vi "1. HelloWorld.vi"() -> ()   [LabVIEW 2011]
panel:
  in  "Disarm":bool
  in  "Arm":bool
  out "OpenSF Error":errorcluster
  out "WriteSF Error":errorcluster
  in  "emergency break":bool
  in  "Destination Id":u16=1
  in  "ServoPositions":T1={"Throttle"=0, "Pitch"=64, "Roll"=64, "Yaw"=64, "Mode"=0, "Data5"=100, "Data6"=100, "Data7"=100}
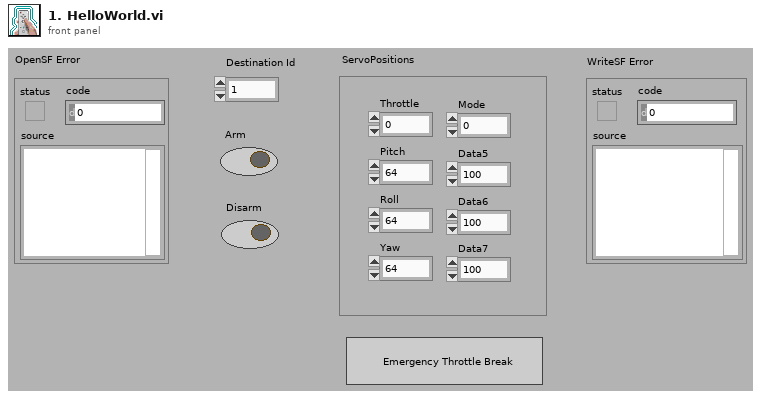
[diagram p1: front panel]
types:
  T1 = cluster{"Throttle":u8, "Pitch":u8, "Roll":u8, "Yaw":u8, "Mode":u8, "Data5":u8, "Data6":u8, "Data7":u8}
  T2 = cluster{"Data0":u8, "Data1":u8, "Data2":u8, "Data3":u8, "Data4":u8, "Data5":u8, "Data6":u8, "Data7":u8}
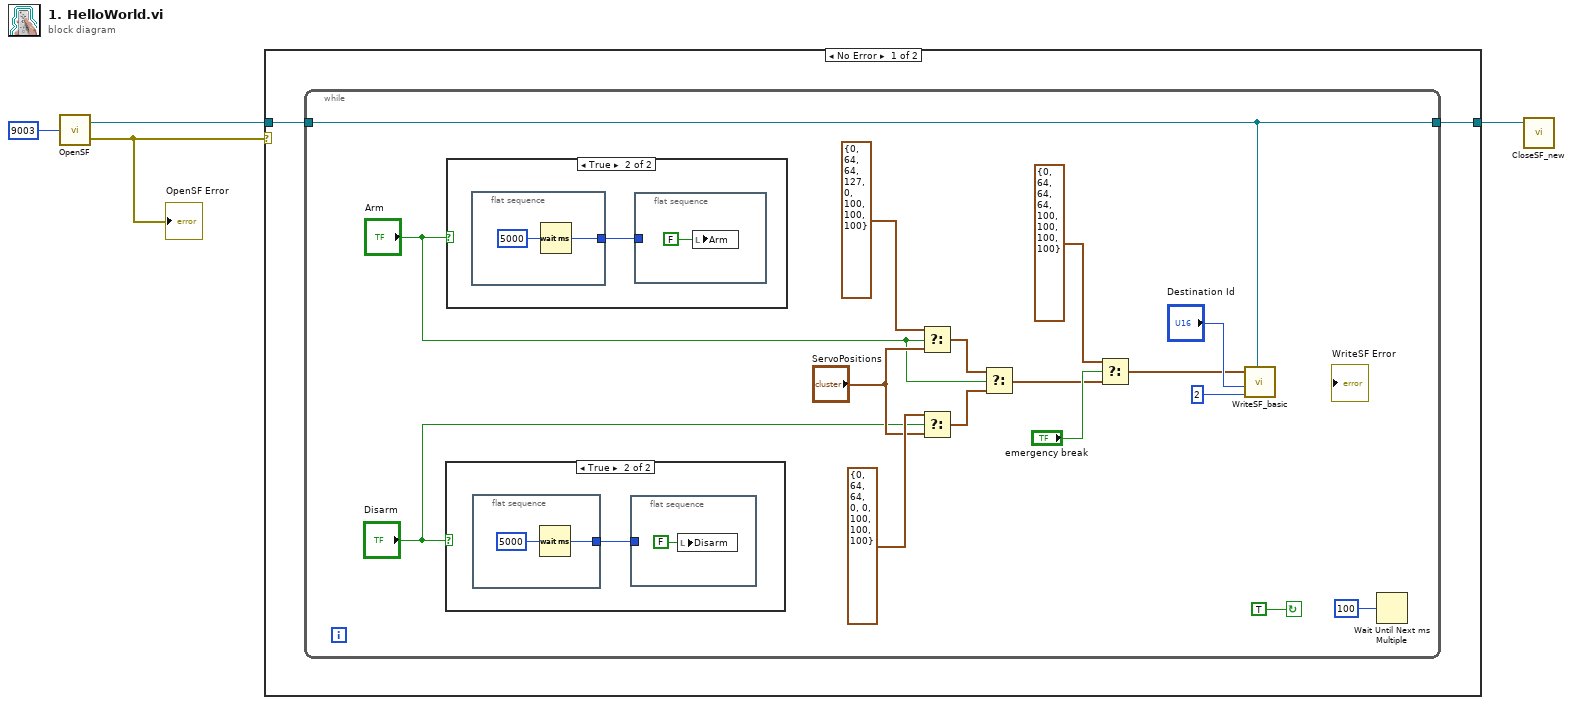
[diagram p0: block diagram]
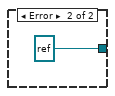
[diagram p4: hidden frame]
diagram:
  n1 = call "OpenSF.vi"("Port number"=u16 9003 ("Port Number")) -> ("connection ID"=w2:refnum<k5>, "Error out"=w3:errorcluster)
  "OpenSF Error" <- w3
  n2 = case shown="No Error" w3 {
    tunnel: w2 -> [w6 _]
    tunnel: [w5 refnum<k5> refnum ("connection ID")] -> w1
    frame No Error {
      n3 = while {
        tunnel: w6 -> [w9]
        tunnel: [w9] -> w5
        stop <- TRUE continue-if-true
        n4 = case shown="True" "Disarm" {
          frame False {
          }
          frame True {
            n5 = flat-sequence {
              tunnel: [w25] -> w23
              frame #0 {
                n6 = Wait (ms)(milliseconds to wait=u32 5000) -> (millisecond timer value=w25:u32)
              }
            }
            n7 = flat-sequence {
              tunnel: w23 -> [_]
              frame #0 {
                n8 = local write "Disarm"(FALSE ("Arm")) -> ()
              }
            }
          }
        }
        n9 = case shown="True" "Arm" {
          frame False {
          }
          frame True {
            n10 = flat-sequence {
              tunnel: [w29] -> w27
              frame #0 {
                n11 = Wait (ms)(milliseconds to wait=u32 5000) -> (millisecond timer value=w29:u32)
              }
            }
            n12 = flat-sequence {
              tunnel: w27 -> [_]
              frame #0 {
                n13 = local write "Arm"(FALSE ("Arm")) -> ()
              }
            }
          }
        }
        n14 = Select(t=T2 {"Data0"=0, "Data1"=64, "Data2"=64, "Data3"=127, "Data4"=0, "Data5"=100, "Data6"=100, "Data7"=100} ("Servo Positions 4"), s="Arm", f="ServoPositions") -> (s? t:f=w16:T1)
        n15 = Select(t=T2 {"Data0"=0, "Data1"=64, "Data2"=64, "Data3"=0, "Data4"=0, "Data5"=100, "Data6"=100, "Data7"=100} ("Servo Positions 4"), s="Disarm", f="ServoPositions") -> (s? t:f=w15:T1)
        n16 = Select(t=w16, s="Arm", f=w15) -> (s? t:f=w12:T1)
        n17 = Select(t=T2 {"Data0"=0, "Data1"=64, "Data2"=64, "Data3"=64, "Data4"=100, "Data5"=100, "Data6"=100, "Data7"=100} ("Servo Positions 4"), s="emergency break", f=w12) -> (s? t:f=w11:T1)
        n18 = call "WriteSF_basic.vi"("Connection ID"=w9, "MsgType"=u8 2, "Destination ID"="Destination Id", "Servo Positions"=w11) -> ()  [unwired: 8 in]
        n19 = Wait Until Next ms Multiple(millisecond multiple=u32 100) -> ()  [unwired: 1 out]
      }
    }
    frame Error {
    }
  }
  n20 = call "CloseSF_new.vi"("connection ID"=w1) -> ()  [unwired: 2 in]
